vi "End Array by Value.vi"(8 "Error In":errorcluster, 11 "Writer In":refnum<class "Writer.lvclass">) -> (0 "Error Out":errorcluster, 3 "Writer Out":refnum<class "Writer.lvclass">)   [LabVIEW 2019, in "LabPack.lvlib" / "Writer.lvclass"]
uses:
  Writer.lvclass
  Writer.lvclass/Writer.ctl
  Public/Status/Read Is Error.vi
  Public/Status/Read Status.vi
  Public/Status/Read Status Message.vi
  Utility/Status Code.vi
  <vilib>/Utility/error.llb/Error Cluster From Error Code.vi
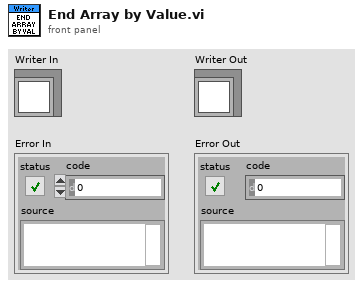
[diagram p1: front panel]
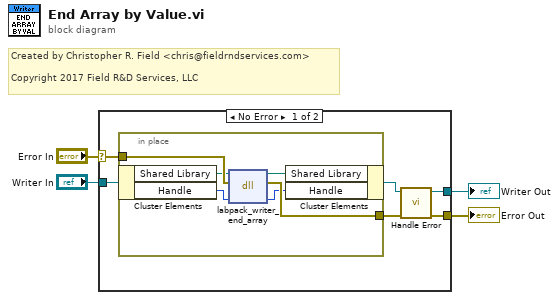
[diagram p0: block diagram]
diagram:
  # "Created by Christopher R. Field <chris@fieldrndservices.com>\n\nCopyright 2017 Field R&D Services, LLC"
  n1 = case shown="No Error" "Error In" {
    selector: "Error In" -> [w10 w18]
    tunnel: [w6 w18] -> w3
    tunnel: "Writer In" -> [w9 w17]
    tunnel: [w5 w17] -> w1
    frame No Error {
      n2 = in-place {
        in-place-border: w10 -> [w16]
        in-place-border: [w15] -> w8
        n3 = in-place-cluster #1(w9) -> ("Shared Library"=w14:path, "Handle"=w13:u64)
        n4 = dll-call lib="D:/Users/cfield/Code/MessagePack/LabPack/LabVIEW/trunk/src/LabPack/Private/labpack-x64.dll" fn="labpack_writer_end_array"(path in=w14, error in=w16, "writer"=w13) -> (path out=w11:path, error out=w15:errorcluster, "writer"=w12:u64)  [unwired: 2 in]
        n5 = in-place-cluster #1("Shared Library"=w11, "Handle"=w12) -> (w7:refnum<class "Writer.lvclass">)
      }
      n6 = call "Handle Error.vi"("Error In"=w8, "Writer In"=w7) -> ("Error Out"=w6:errorcluster, "Writer Out"=w5:refnum<class "Writer.lvclass">)  [unwired: 8 in]
    }
    frame Error {
    }
  }
  "Error Out" <- w3
  "Writer Out" <- w1
